vi "Write AIP.vi"(8 "error in (no error)":errorcluster, 10 "AIP Command":T1, 11 "AIP Deploy Command in":refnum<class "AIP Command.lvclass">) -> (0 "error out":errorcluster, 3 "AIP Deploy Command out":refnum<class "AIP Command.lvclass">)   [LabVIEW 2015, in "RDS Child Messages.lvlib" / "AIP Command.lvclass"]
uses:
  RDS Framework/RDS Message Class/AIP Command.lvclass
  RDS Framework/RDS Message Class/AIP Command Control.ctl
  RDS Framework/RDS Message Class/AIP Command.lvclass/AIP Command.ctl
  RDS Child Messages.lvlib
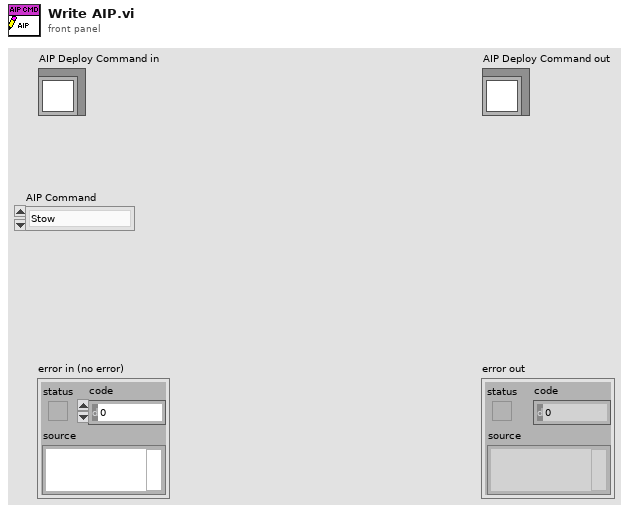
[diagram p1: front panel]
types:
  T1 = typedef "RDS Child Messages.lvlib/AIP Command Control.ctl" = enum16{"Stow", "Deploy", "Stop", "Validate Sensors", "Jog Deploy FP", "Jog Stow FP", "Jog Deploy FS", "Jog Stow FS", "Jog Deploy AP", "Jog Stow AP", "Jog Deploy AS", "Jog Stow AS", "Deploy FP", "Deploy FS", "Deploy AP", "Deploy AS", "Stow FP", "Stow FS", "Stow AP", "Stow AS"}
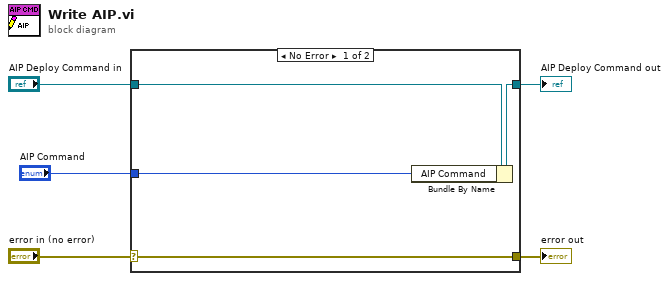
[diagram p0: block diagram]
diagram:
  n1 = case shown="No Error" "error in (no error)" {
    selector: "error in (no error)" -> [w9 w10]
    tunnel: [w9 w10] -> w4
    tunnel: [w7 w11] -> w2
    tunnel: "AIP Deploy Command in" -> [w8 w11]
    tunnel: "AIP Command" -> [w6 _]
    frame No Error {
      n2 = Bundle By Name(cluster=w8, "AIP Command"=w6) -> (w7:refnum<class "AIP Command.lvclass">)
    }
    frame Error {
    }
  }
  "error out" <- w4
  "AIP Deploy Command out" <- w2
